vi "Com_SECS Equipment _Timeout Setting.vi"(6 "Method":enum16{"Get", "Put"}(ring), 8 "error in":errorcluster, 10 "Timeout Setting In":T1={"T3(Reply Timeout)"=45.0, "T5(Separation Timeout)"=10.0, "T6(Control Timeout)"=5.0, "T7(Not Selected Timeout)"=10.0, "T8(Inter-Character Timeout)"=5.0}, 11 "Buffer Data In":T2) -> (0 "error out":errorcluster, 2 "Timeout Setting Out":T1={"T3(Reply Timeout)"=45.0, "T5(Separation Timeout)"=10.0, "T6(Control Timeout)"=5.0, "T7(Not Selected Timeout)"=10.0, "T8(Inter-Character Timeout)"=5.0}, 3 "Buffer Data Out":T2)   [LabVIEW 2016]
uses:
  Data Def/Com_SECS Equipment _Buffer Data.ctl
  Data Def/Com_SECS Equipment _Connection Setting.ctl
  Data Def/Com_SECS Equipment _Timeout Setting.ctl
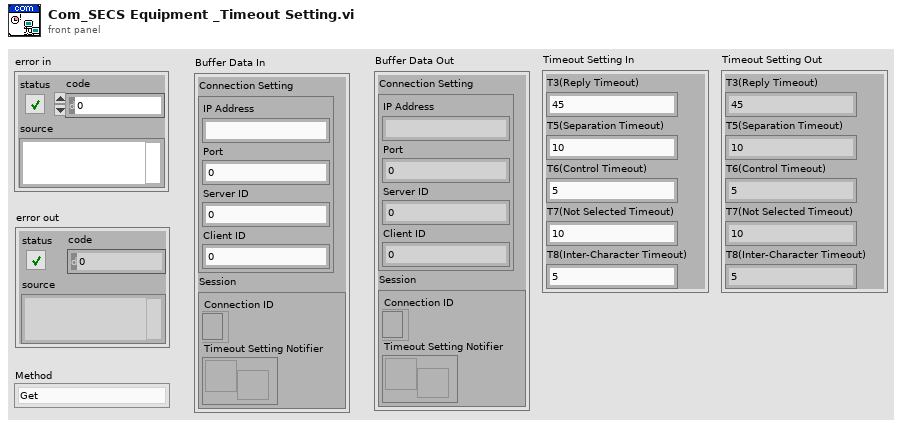
[diagram p1: front panel]
types:
  T1 = typedef "Com_SECS Equipment _Timeout Setting.ctl" = cluster{"T3(Reply Timeout)":dbl, "T5(Separation Timeout)":dbl, "T6(Control Timeout)":dbl, "T7(Not Selected Timeout)":dbl, "T8(Inter-Character Timeout)":dbl}
  T2 = typedef "Com_SECS Equipment _Buffer Data.ctl" = cluster{"Connection Setting":T3, "Session":cluster{"Connection ID":refnum<k5>, "Timeout Setting Notifier":refnum<notifier>}}
  T3 = typedef "Com_SECS Equipment _Connection Setting.ctl" = cluster{"IP Address":string, "Port":u16, "Server ID":u16, "Client ID":u16}
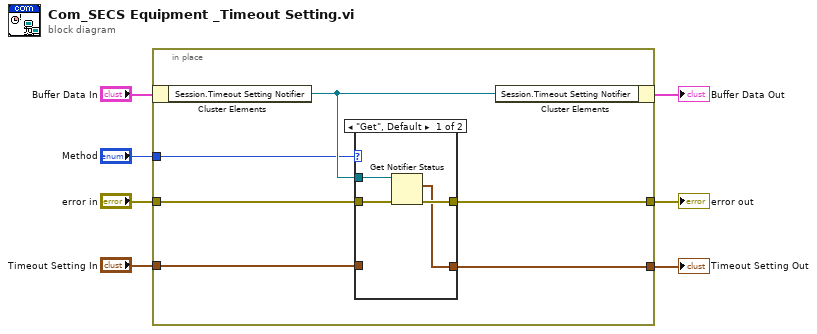
[diagram p0: block diagram]
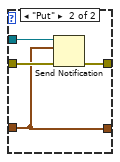
[diagram p2: hidden frame]
diagram:
  n1 = in-place {
    in-place-border: "error in" -> [w12]
    in-place-border: "Timeout Setting In" -> [w11]
    in-place-border: [w10] -> w3
    in-place-border: "Method" -> [w9]
    in-place-border: [w8] -> w1
    n2 = in-place-cluster #1("Buffer Data In") -> ("Session.Timeout Setting Notifier"=w13:refnum<notifier>)
    n3 = case shown="\"Get\", Default" w9 {
      tunnel: w13 -> [w16 w21]
      tunnel: w12 -> [w17 w20]
      tunnel: w11 -> [_ w18]
      tunnel: [w15 w19] -> w10
      tunnel: [w14 w18] -> w8
      frame "Get", Default {
        n4 = Get Notifier Status(notifier=w16, error in (no error)=w17) -> (current notification=w14:T1, error out=w15:errorcluster)  [unwired: 3 out]
      }
      frame "Put" {
        n5 = Send Notification(notification=w18, notifier=w21, error in (no error)=w20) -> (error out=w19:errorcluster)  [unwired: 1 out]
      }
    }
    n6 = in-place-cluster #1("Session.Timeout Setting Notifier"=w13) -> (→"Buffer Data Out":T2)
  }
  "error out" <- w3
  "Timeout Setting Out" <- w1
